vi "公式复合写入.vi"(8 "公式":cluster{"X^2":dbl, "X":dbl, "b":dbl}, 9 "量程下拉列表":enum16{"低量程", "高量程"}(ring), 10 "测量模式":T1(ring), 11 "参数下拉列表":u16(ring) items=["总氮"=2]) -> ()   [LabVIEW 2016, in "斯坦道通用流路CODmn.lvlib"]
uses:
  <vilib>/Utility/miscctls.llb/LVPointTypeDef.ctl
panel:
  in  "读取":bool
  in  "一键写入":bool=TRUE
  out "连接的字符串":string
  in  "关闭":bool
  in  "写入":bool
  # "请选择要写入的参数"
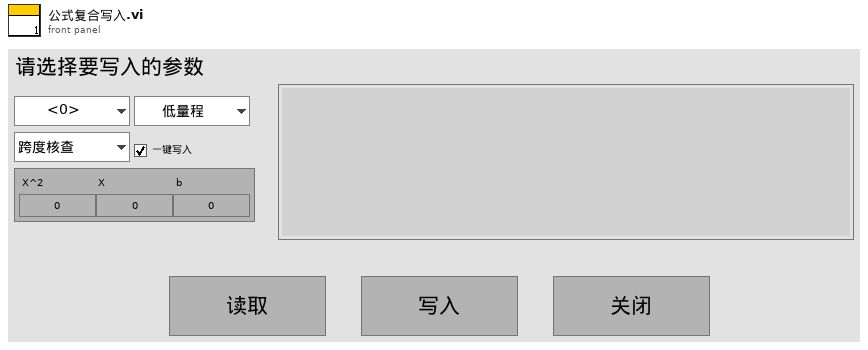
[diagram p1: front panel]
types:
  T1 = enum16{"跨度核查", "水样测量", "零点核查", "标样核查", "加标回收", "快捷测试", "空白校准", "标样校准"}
  T2 = typedef "LVPointTypeDef.ctl" = cluster{"Horizontal":i16, "Vertical":i16}
  T3 = cluster{"系统时间":timestamp, "工作状态":u16, "测量模式":enum16{"待机", "连续模式", "周期模式", "定点模式", "受控模式", "手动模式"}, "告警代码":u16, "故障代码":u16, "日志代码":u16, "软件版本":u16, "F0":sgl, "F1":sgl, "F2":sgl, "F3":sgl, "T":sgl, "H":sgl, "id":u16, "flowid":u16, "量程":u16, "总磷控温温度1":sgl, "营养盐控温温度2":sgl, "ADC":sgl}
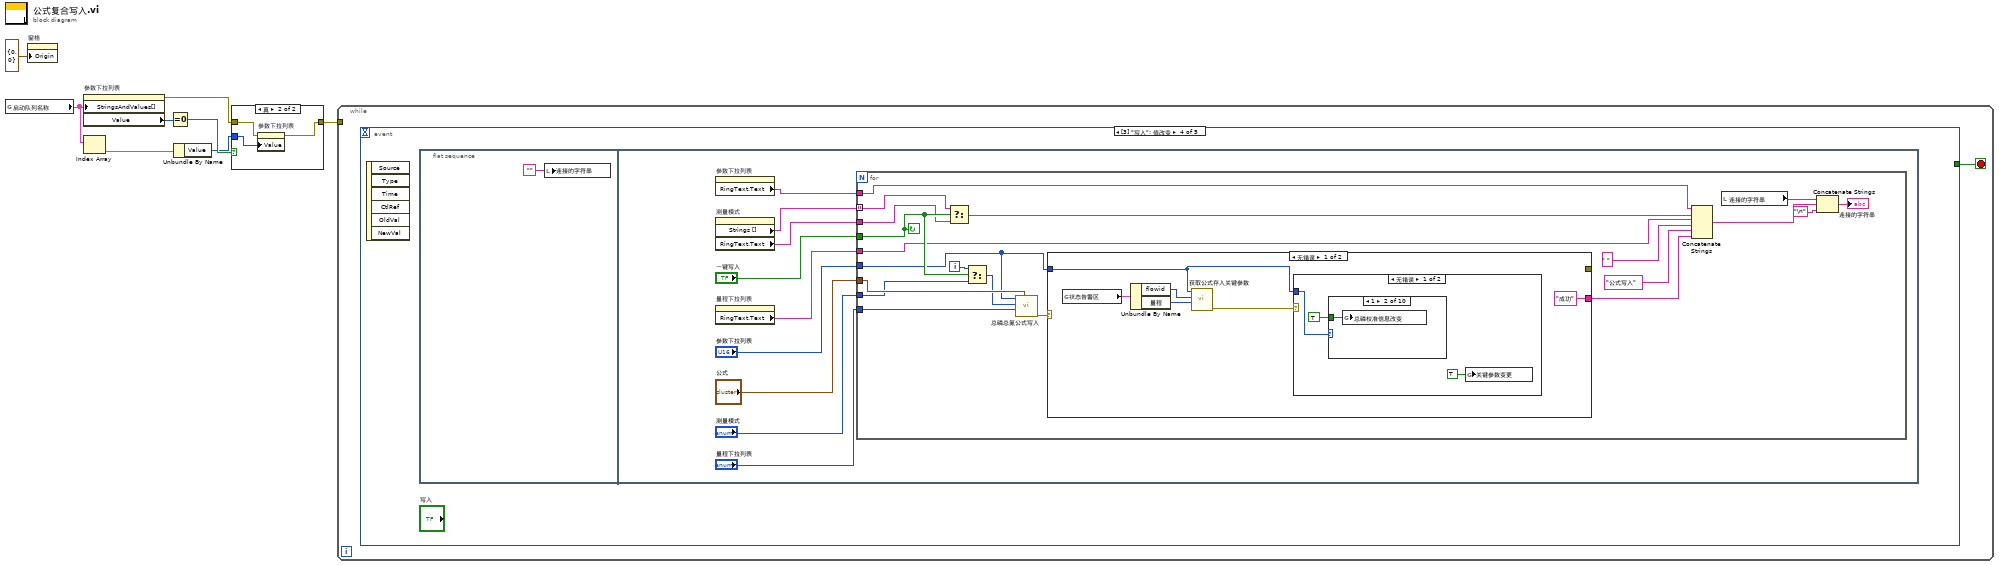
[diagram p0: block diagram]
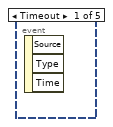
[diagram p3: hidden frame]
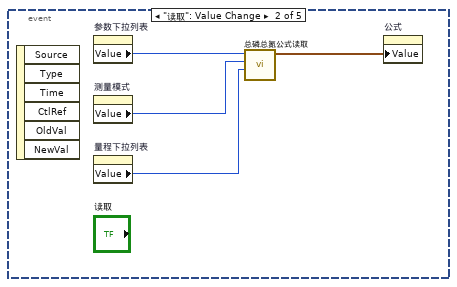
[diagram p4: hidden frame]
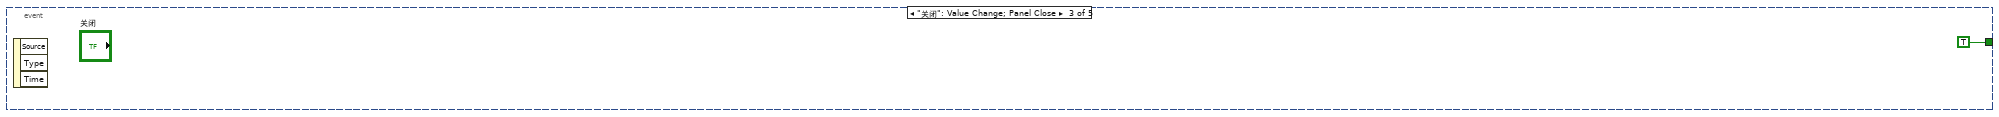
[diagram p5: hidden frame]
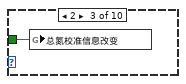
[diagram p7: hidden frame]
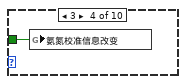
[diagram p8: hidden frame]
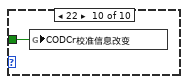
[diagram p14: hidden frame]
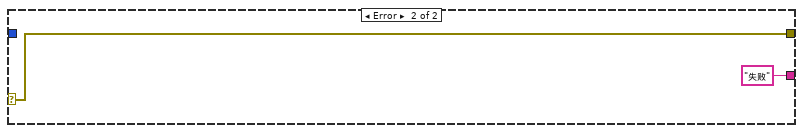
[diagram p16: hidden frame]
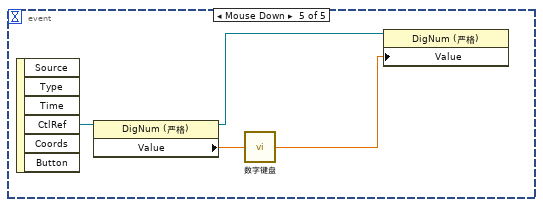
[diagram p17: hidden frame]
diagram:
  n1 = global read "model config var.vi" "启动队列名称"() -> (w3:cluster{"String":string, "Value":u16}[])
  n2 = property on="窗格" class="Pane"("Origin"=T2 {"Horizontal"=0, "Vertical"=0} ("原点")) -> ()  [unwired: 2 in, 2 out]
  n3 = property on="参数下拉列表" class="Ring (严格)"("StringsAndValues[]"=w3) -> (error out=w5:errorcluster, "Value"=w4:u16)  [unwired: 2 in, 1 out]
  n4 = Index Array(array=w3) -> (element=w2:cluster{"String":string, "Value":u16})  [unwired: 1 in]
  n5 = Equal To 0?(x=w4) -> (x = 0?=w7:bool)
  n6 = Unbundle By Name(w2) -> ("Value"=w6:u16)
  n7 = case shown="真" w7 {
    tunnel: w5 -> [w9 w12]
    tunnel: [w9 w11] -> w1
    tunnel: w6 -> [_ w10]
    frame False {
    }
    frame True {
      n8 = property on="参数下拉列表" class="Ring (严格)"(error in=w12, "Value"=w10) -> (error out=w11:errorcluster)  [unwired: 1 in, 1 out]
    }
  }
  n9 = while {
    tunnel: w1 -> [_]
    stop <- w13 stop-if-true
    n10 = event shown="[3] \"写入\": 值改变" {
      selector: _ -> [_ _ _ _ _]
      dyn-events: _ -> [_ _ _ _ _]
      timeout: _ -> [_ _ _ _ _]
      tunnel: [_ _ TRUE _ _] -> w13
      event Timeout {
        n11 = event-data() -> ()  [unwired: 1 in, 3 out]
      }
      event "读取": Value Change {
        n12 = event-data() -> ()  [unwired: 1 in, 6 out]
        n13 = property on="参数下拉列表" class="Ring (严格)"() -> ("Value"=w17:u16)  [unwired: 2 in, 2 out]
        n14 = property on="测量模式" class="Enum (严格)"() -> ("Value"=w16:T1)  [unwired: 2 in, 2 out]
        n15 = property on="量程下拉列表" class="Enum (严格)"() -> ("Value"=w15:enum16{"低量程", "高量程"})  [unwired: 2 in, 2 out]
        n16 = call "总磷总氮公式读取.vi"("量程"=w15, "测量模式"=w16, "测量参数"=w17) -> ("公式"=w14:cluster{"X^2":dbl, "X":dbl, "b":dbl})  [unwired: 7 in, 1 out]
        n17 = property on="公式" class="Clust (严格)"("Value"=w14) -> ()  [unwired: 2 in, 2 out]
      }
      event "关闭": Value Change; Panel Close {
        n18 = event-data() -> ()  [unwired: 1 in, 3 out]
      }
      event "写入": Value Change {
        n19 = event-data() -> ()  [unwired: 1 in, 6 out]
        n20 = flat-sequence {
          frame #0 {
            n21 = local write "连接的字符串"("") -> ()
          }
          frame #1 {
            n22 = property on="参数下拉列表" class="Ring (严格)"() -> ("RingText.Text"=w21:string)  [unwired: 2 in, 2 out]
            n23 = property on="测量模式" class="Enum (严格)"() -> ("Strings []"=w25:string[], "RingText.Text"=w24:string)  [unwired: 2 in, 2 out]
            n24 = property on="量程下拉列表" class="Enum (严格)"() -> ("RingText.Text"=w20:string)  [unwired: 2 in, 2 out]
            n25 = for {
              tunnel: "公式" -> [w48]
              tunnel: "参数下拉列表" -> [w29]
              tunnel: "量程下拉列表" -> [w47]
              tunnel: w25 -> [w41] mode=indexing
              tunnel: w24 -> [w40]
              tunnel: "一键写入" -> [w42]
              tunnel: "测量模式" -> [w44]
              tunnel: w21 -> [w32]
              tunnel: w20 -> [w30]
              i -> [w45]
              stop <- w42 continue-if-true
              n26 = Select(t=w41, s=w42, f=w40) -> (s? t:f=w34:string)
              n27 = Select(t=w45, s=w42, f=w44) -> (s? t:f=w43:i32)
              n28 = call "总磷总氮公式写入.vi"("公式"=w48, "量程"=w47, "测量模式"=w43, "测量参数"=w29) -> ("error out"=w46:errorcluster)  [unwired: 7 in]
              n29 = case shown="无错误" w46 {
                selector: w46 -> [_ w63]
                tunnel: [_ w63] -> _
                tunnel: ["成功" "失败"] -> w33
                tunnel: w29 -> [w50 _]
                frame No Error {
                  n30 = global read "VAR总磷总氮全局变量.vi" "状态告警区"() -> (w51:T3)
                  n31 = Unbundle By Name(w51) -> ("flowid"=w53:u16, "量程"=w52:u16)
                  n32 = call "获取公式存入关键参数.vi"("量程"=w52, "flowid"=w53, "id"=w50) -> ("error out"=w49:errorcluster)  [unwired: 7 in, 1 out]
                  n33 = case shown="无错误" w49 {
                    tunnel: w50 -> [w55 _]
                    frame No Error {
                      n34 = case shown="1" w55 {
                        tunnel: TRUE ("总磷关键参数改变") -> [_ w58 w59 w60 _ _ _ _ _ w61]
                        frame 0, Default {
                        }
                        frame 1 {
                          n35 = global write "VAR总磷总氮全局变量.vi" "总磷校准信息改变"(w58) -> ()
                        }
                        frame 2 {
                          n36 = global write "VAR总磷总氮全局变量.vi" "总氮校准信息改变"(w59) -> ()
                        }
                        frame 3 {
                          n37 = global write "VAR总磷总氮全局变量.vi" "氨氮校准信息改变"(w60) -> ()
                        }
                        frame 4 {
                        }
                        frame 5 {
                        }
                        frame 6 {
                        }
                        frame 7 {
                        }
                        frame 8 {
                        }
                        frame 22 {
                          n38 = global write "VAR总磷总氮全局变量.vi" "CODCr校准信息改变"(w61) -> ()
                        }
                      }
                      n39 = global write "VAR总磷总氮全局变量.vi" "关键参数变更"(TRUE ("关键参数变更")) -> ()
                    }
                    frame Error {
                    }
                  }
                }
                frame Error {
                }
              }
              n40 = Concatenate Strings(w32, w34, w30, " " ("字符串"), "公式写入", w33) -> (w38:string)
              n41 = local read "连接的字符串"() -> (w35:string)
              n42 = Concatenate Strings(w35, w38, "\n") -> (→"连接的字符串":string)
            }
          }
        }
      }
      event "公式.X^2", "公式.X", "公式.b": Mouse Down {
        n43 = event-data() -> ("CtlRef"=w67:refnum<vi>)  [unwired: 1 in, 5 out]
        n44 = property class="DigNum (严格)"(reference=w67) -> (reference out=w64:refnum<vi>, "Value"=w66:dbl)  [unwired: 1 in, 1 out]
        n45 = call "数字键盘.vi"("OldNumber"=w66) -> ("NewNumber"=w65:dbl)
        n46 = property class="DigNum (严格)"(reference=w64, "Value"=w65) -> ()  [unwired: 1 in, 2 out]
      }
    }
  }
